vi "R1SBRControl_2.vi"(8 "error constant":errorcluster, 11 "LabVIEW Web Service":refnum<class "Web Service.lvclass">) -> (0 "error out":errorcluster)   [LabVIEW 2016]
uses:
  <vilib>/wsapi/Web Service.lvclass
  R1Controls/R1SBR_SetParams.ctl
  <vilib>/Utility/Variable/NI_VariableUtilities.lvlib
panel:
  out "Numeric 2":i32
  out "current time":timestamp
  out "No phases":i32
  out "Numeric":i32
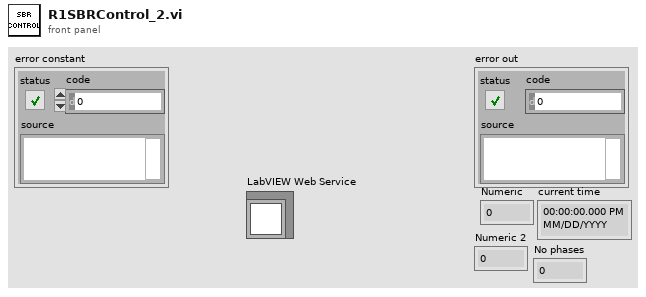
[diagram p1: front panel]
types:
  T1 = cluster{"Media Pump":bool, "Water Pump":bool, "Gas Pump":bool, "Effluent Pump":bool}
  T2 = typedef "R1SBR_SetParams.ctl" = cluster{"Phase":string, "Time, min":dbl, "SBR_Manual":cluster{"Media Pump":bool, "Water Pump":bool, "Gas Pump":bool, "Effluent Pump":bool}}[]
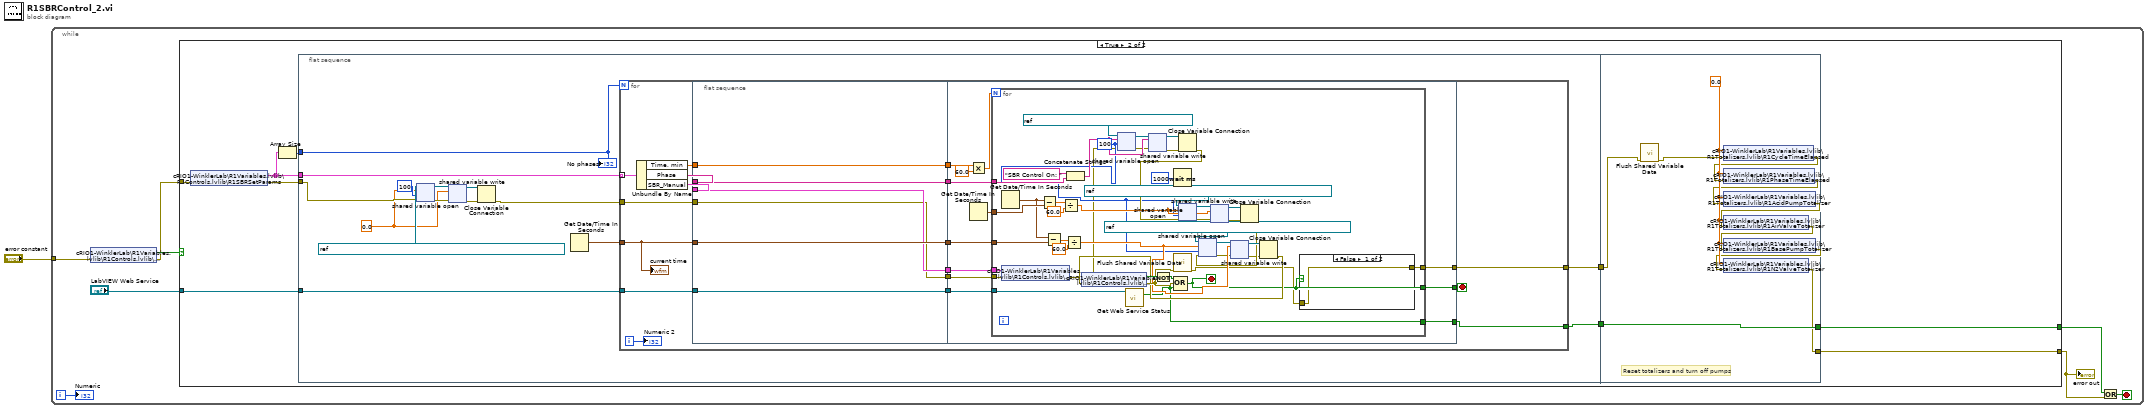
[diagram p0: block diagram]
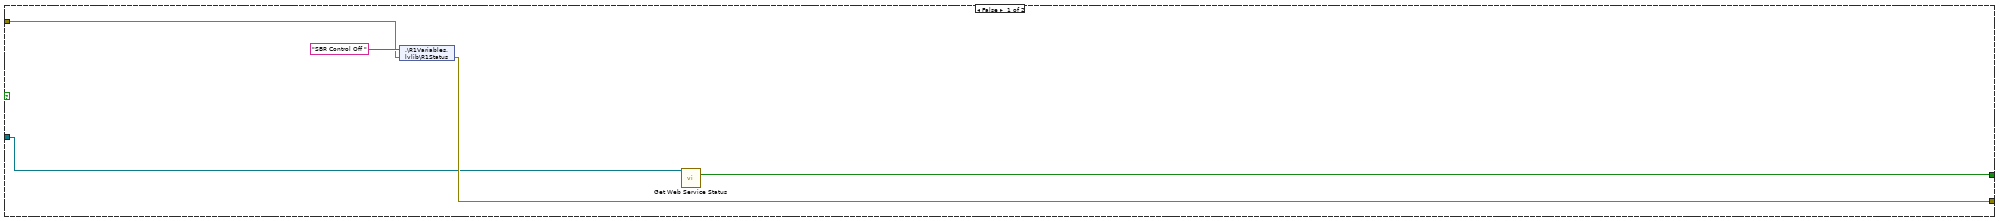
[diagram p2: hidden frame]
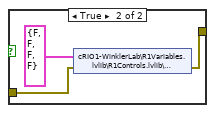
[diagram p3: hidden frame]
diagram:
  n1 = while {
    tunnel: "error constant" -> [w8]
    i -> [w3]
    stop <- w4 stop-if-true
    n2 = shared-variable "cRIO1-WinklerLab\\R1Variables.lvlib\\R1Controls.lvlib\\R1SBRSwitch"(error in=w8) -> (w9:bool, error out=w7:errorcluster)
    n3 = case shown="True" w9 {
      tunnel: "LabVIEW Web Service" -> [w11 w21]
      tunnel: w7 -> [w13 w20]
      tunnel: [w12 w15] -> w5
      tunnel: [w10 w17] -> w2
      frame False {
        n4 = shared-variable ".\\R1Variables.lvlib\\R1Status"("SBR Control Off " ("string"), error in=w13) -> (error out=w12:errorcluster)
        n5 = call <vilib>:"Get Web Service Status.vi"("LabVIEW Web Service"=w11) -> ("service stopping?"=w10:bool)  [unwired: 12 in, 2 out]
      }
      frame True {
        n6 = shared-variable "cRIO1-WinklerLab\\R1Variables.lvlib\\R1Controls.lvlib\\R1SBRSetParams"(error in=w20) -> (w22:T2, error out=w19:errorcluster)
        n7 = Array Size(array=w22) -> (size(s)=w23:i32)
        n8 = flat-sequence {
          tunnel: w22 -> [w37]
          tunnel: w23 -> [w38]
          tunnel: w21 -> [w36]
          tunnel: w19 -> [w27]
          tunnel: [w34] -> w18
          tunnel: [w24] -> w16
          tunnel: w18 -> [w124]
          tunnel: [w122] -> w17
          tunnel: w16 -> [w122]
          tunnel: [w121] -> w15
          frame #0 {
            w25 = 0.0 ("R1CycleTimeElapsed")
            n9 = shared-variable-open(refnum<k21> "ni.var.psp://crio1-winklerlab/R1Variables/R1Totalizers/R1CycleTimeElapsed" ("shared variable refnum in"), w27, w25, 100 ("timeout ms")) -> (w32:refnum<k21>, w30:errorcluster)  [unwired: 2 in]
            n10 = shared-variable-write(w32, w30, w25) -> (w31:refnum<k21>, w29:errorcluster)
            n11 = Close Variable Connection(8:w29, 11:w31) -> (0:w26:errorcluster)
            n12 = Get Date/Time In Seconds() -> (seconds since 1Jan1904=w35:timestamp)
            n13 = for {
              N: w38 -> [_]
              tunnel: w37 -> [w55] mode=indexing
              tunnel: w36 -> [w53]
              tunnel: w26 -> [w47]
              tunnel: [w45] -> w34
              tunnel: w35 -> [w42]
              tunnel: [w41] -> w24
              i -> [w43]
              stop <- w44 stop-if-true
              n14 = Unbundle By Name(w55) -> ("Time, min"=w50:dbl, "Phase"=w49:string, "SBR_Manual"=w54:T1)
              n15 = flat-sequence {
                tunnel: w50 -> [w60]
                tunnel: w54 -> [w57]
                tunnel: w53 -> [w61]
                tunnel: [w61] -> w52
                tunnel: [w60] -> w51
                tunnel: w49 -> [w59]
                tunnel: [w59] -> w48
                tunnel: w47 -> [w56]
                tunnel: w42 -> [w58]
                tunnel: [w58] -> w46
                tunnel: [w57] -> w40
                tunnel: [w56] -> w39
                tunnel: [w72] -> w44
                tunnel: w52 -> [w73]
                tunnel: w51 -> [w71]
                tunnel: w48 -> [w68]
                tunnel: w46 -> [w66]
                tunnel: [w65] -> w45
                tunnel: [w64] -> w41
                tunnel: w40 -> [w63]
                tunnel: w39 -> [w62]
                frame #0 {
                }
                frame #1 {
                  n16 = Get Date/Time In Seconds() -> (seconds since 1Jan1904=w67:timestamp)
                  n17 = Multiply(x=w71, y=60.0) -> (x*y=w69:dbl)
                  n18 = for {
                    N: w69 -> [_]
                    tunnel: w73 -> [w106]
                    tunnel: [w76] -> w72
                    tunnel: w68 -> [w113]
                    tunnel: w67 -> [w110]
                    tunnel: w66 -> [w107]
                    tunnel: [w74] -> w65
                    tunnel: [w80] -> w64
                    tunnel: w63 -> [w79]
                    tunnel: w62 -> [w78]
                    stop <- w76 stop-if-true
                    w81 = 100 ("timeout ms")
                    n19 = Get Date/Time In Seconds() -> (seconds since 1Jan1904=w108:timestamp)
                    n20 = shared-variable "cRIO1-WinklerLab\\R1Variables.lvlib\\R1Controls.lvlib\\R1SBRManual"(w79, error in=w78) -> (error out=w77:errorcluster)
                    n21 = Subtract(x=w108, y=w110) -> (x-y=w111:dbl)
                    n22 = Subtract(x=w108, y=w107) -> (x-y=w105:dbl)
                    n23 = Divide(x=w111, y=60.0) -> (x/y=w89:dbl)
                    n24 = Divide(x=w105, y=60.0) -> (x/y=w98:dbl)
                    n25 = Concatenate Strings("SBR Control On: " ("string"), w113) -> (w85:string)
                    n26 = shared-variable-open(refnum<k21> "ni.var.psp://crio1-winklerlab/R1Variables/R1Status" ("shared variable refnum in"), w77, w85, w81) -> (w87:refnum<k21>, w84:errorcluster)  [unwired: 2 in]
                    n27 = call <vilib>:"Get Web Service Status.vi"("LabVIEW Web Service"=w106) -> ("service stopping?"=w80:bool)  [unwired: 12 in, 2 out]
                    n28 = shared-variable-write(w87, w84, w85) -> (w88:refnum<k21>, w83:errorcluster)
                    n29 = Wait (ms)(milliseconds to wait=u32 1000) -> ()  [unwired: 1 out]
                    n30 = Close Variable Connection(8:w83, 11:w88) -> (0:w82:errorcluster)
                    n31 = shared-variable-open(refnum<k21> "ni.var.psp://crio1-winklerlab/R1Variables/R1Totalizers/R1PhaseTimeElapsed" ("shared variable refnum in"), w82, w89, w81) -> (w96:refnum<k21>, w94:errorcluster)  [unwired: 2 in]
                    n32 = shared-variable-write(w96, w94, w89) -> (w97:refnum<k21>, w93:errorcluster)
                    n33 = Close Variable Connection(8:w93, 11:w97) -> (0:w92:errorcluster)
                    n34 = shared-variable-open(refnum<k21> "ni.var.psp://crio1-winklerlab/R1Variables/R1Totalizers/R1CycleTimeElapsed" ("shared variable refnum in"), w92, w98, w81) -> (w101:refnum<k21>, w91:errorcluster)  [unwired: 2 in]
                    n35 = shared-variable-write(w101, w91, w98) -> (w102:refnum<k21>, w90:errorcluster)
                    n36 = Close Variable Connection(8:w90, 11:w102) -> (0:w99:errorcluster)
                    n37 = shared-variable "cRIO1-WinklerLab\\R1Variables.lvlib\\R1Controls.lvlib\\R1SBRSwitch"(error in=w99) -> (w116:bool, error out=w103:errorcluster)
                    n38 = Not(x=w116) -> (.not. x?=w115:bool)
                    n39 = call <vilib>:"Flush Shared Variable Data.vi"("error in (no error)"=w103) -> ("error out"=w75:errorcluster)  [unwired: 10 in]
                    n40 = Compound Arithmetic op=OR(w115, w103, w80) -> (w76:bool)
                    n41 = case shown="False" w76 {
                      tunnel: w75 -> [w117 w119]
                      tunnel: [w117 w118] -> w74
                      frame False {
                      }
                      frame True {
                        n42 = shared-variable "cRIO1-WinklerLab\\R1Variables.lvlib\\R1Controls.lvlib\\R1SBRManual"(T1 {"Media Pump"=FALSE, "Water Pump"=FALSE, "Gas Pump"=FALSE, "Effluent Pump"=FALSE} ("R1SBR_Manual"), error in=w119) -> (error out=w118:errorcluster)
                      }
                    }
                  }
                }
              }
              "Numeric 2" <- w43
              "current time" <- w42
            }
            "No phases" <- w38
          }
          frame #1 {
            w130 = 0.0 ("R1CycleTimeElapsed")
            # "Reset totalizers and turn off pumps"
            n43 = call <vilib>:"Flush Shared Variable Data.vi"("error in (no error)"=w124) -> ("error out"=w123:errorcluster)  [unwired: 10 in]
            n44 = shared-variable "cRIO1-WinklerLab\\R1Variables.lvlib\\R1Totalizers.lvlib\\R1CycleTimeElapsed"(w130, error in=w123) -> (error out=w129:errorcluster)
            n45 = shared-variable "cRIO1-WinklerLab\\R1Variables.lvlib\\R1Totalizers.lvlib\\R1PhaseTimeElapsed"(w130, error in=w129) -> (error out=w128:errorcluster)
            n46 = shared-variable "cRIO1-WinklerLab\\R1Variables.lvlib\\R1Totalizers.lvlib\\R1AcidPumpTotalizer"(w130, error in=w128) -> (error out=w127:errorcluster)
            n47 = shared-variable "cRIO1-WinklerLab\\R1Variables.lvlib\\R1Totalizers.lvlib\\R1AirValveTotalizer"(w130, error in=w127) -> (error out=w126:errorcluster)
            n48 = shared-variable "cRIO1-WinklerLab\\R1Variables.lvlib\\R1Totalizers.lvlib\\R1BasePumpTotalizer"(w130, error in=w126) -> (error out=w125:errorcluster)
            n49 = shared-variable "cRIO1-WinklerLab\\R1Variables.lvlib\\R1Totalizers.lvlib\\R1N2ValveTotalizer"(w130, error in=w125) -> (error out=w121:errorcluster)
          }
        }
      }
    }
    "error out" <- w5
    n50 = Or(x=w2, y=w5) -> (x .or. y?=w4:bool)
    "Numeric" <- w3
  }
